vi "Keithley2100.ProcCases.vi"(0 "i ref in":refnum<vi>, 1 "selector":string, 2 "Data":T1, 3 "call cluster":T2={"Object"="", "Selector"="", "CallType"=enum."synchronous", "Async Object"="", "Async Selector"="", "Data Descriptor"="", "Data"=[], "Error #"=0, "Expire"=0}, 5 "error in (no error)":errorcluster) -> (14 "i ref out":refnum<vi>, 17 "answer cluster":T2={"Object"="", "Selector"="", "CallType"=enum."synchronous", "Async Object"="", "Async Selector"="", "Data Descriptor"="", "Data"=[], "Error #"=0, "Expire"=0}, 19 "error out":errorcluster)   [LabVIEW 2014, in "Keithley2100.lvlib"]
doc: "This method is called by a process from within the default case in the event loop. The methods of a class that are linked to events will be called from THIS method. Add your code here."
uses:
  Keithley2100.lvlib
  CS_Core/CSSystem/CoreDefs/CoreDefs.call_type.ctl
  CS_Core/BaseProcess/BaseProcess.descriptor string definition.ctl
  CS_Core/CSSystem/CoreDefs/CoreDefs.rawDataType.ctl
  CS_Core/CSSystem/CoreLib/CoreLib.string 2 byte array.vi
  CS_Core/CSSystem/CoreLib/CoreLib.double 2 byte array.vi
  CS_Core/CSSystem/CoreLib/CoreLib.byte array 2 int.vi
  CS_Core/CSSystem/CoreLib/CoreLib.byte array 2 double.vi
  CS_Core/CSSystem/CoreLib/CoreLib.lvlib
  CS_Core/BaseProcess/BaseProcess.lvlib
  CS_Core/CSApplicationBaseClasses/DeviceBase/DeviceBase.lvlib
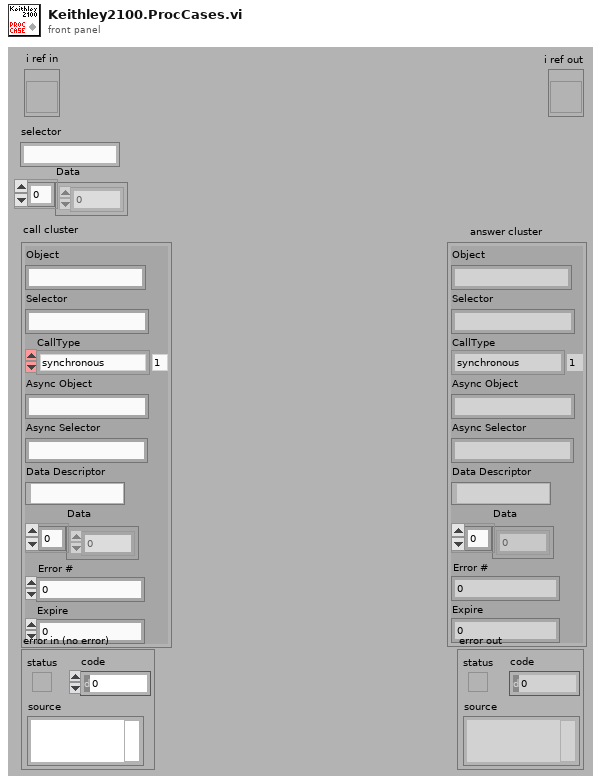
[diagram p1: front panel]
types:
  T1 = typedef "CoreDefs.rawDataType.ctl" = i8[]
  T2 = typedef "CoreDefs.call_type.ctl" = cluster{"Object":string, "Selector":string, "CallType":enum16{"simple", "synchronous", "asynchronous"}, "Async Object":string, "Async Selector":string, "Data Descriptor":T3, "Data":T1, "Error #":i32, "Expire":u32}
  T3 = typedef "BaseProcess.lvlib/BaseProcess.descriptor string definition.ctl" = string
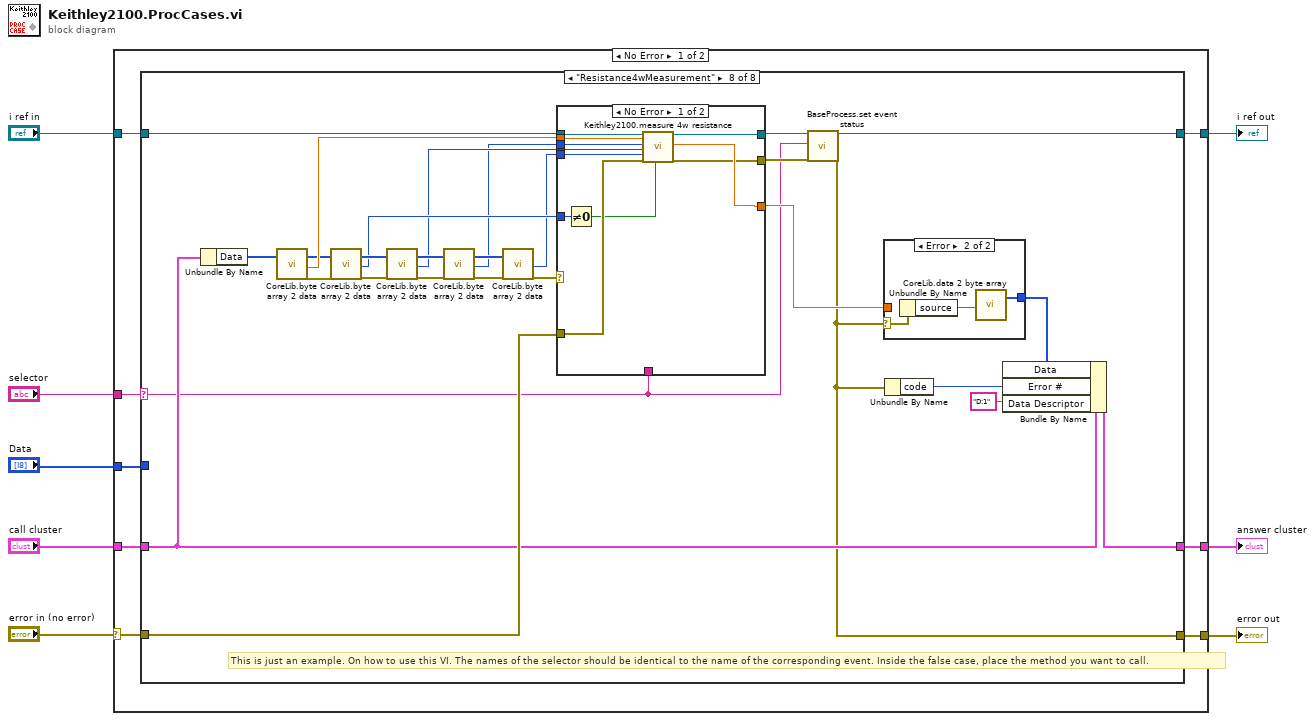
[diagram p0: block diagram]
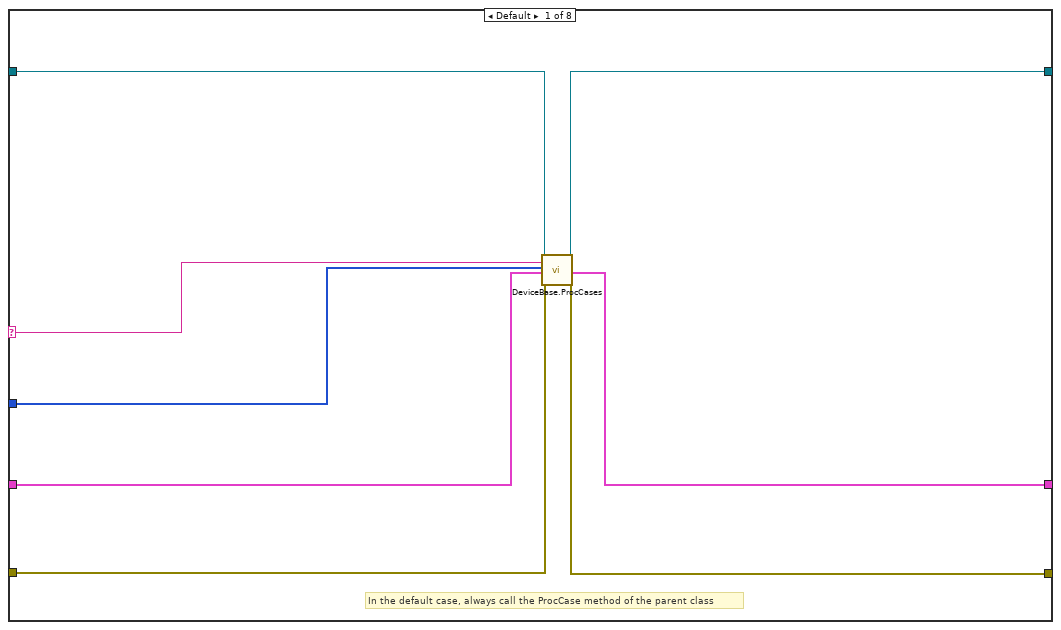
[diagram p2: hidden frame]
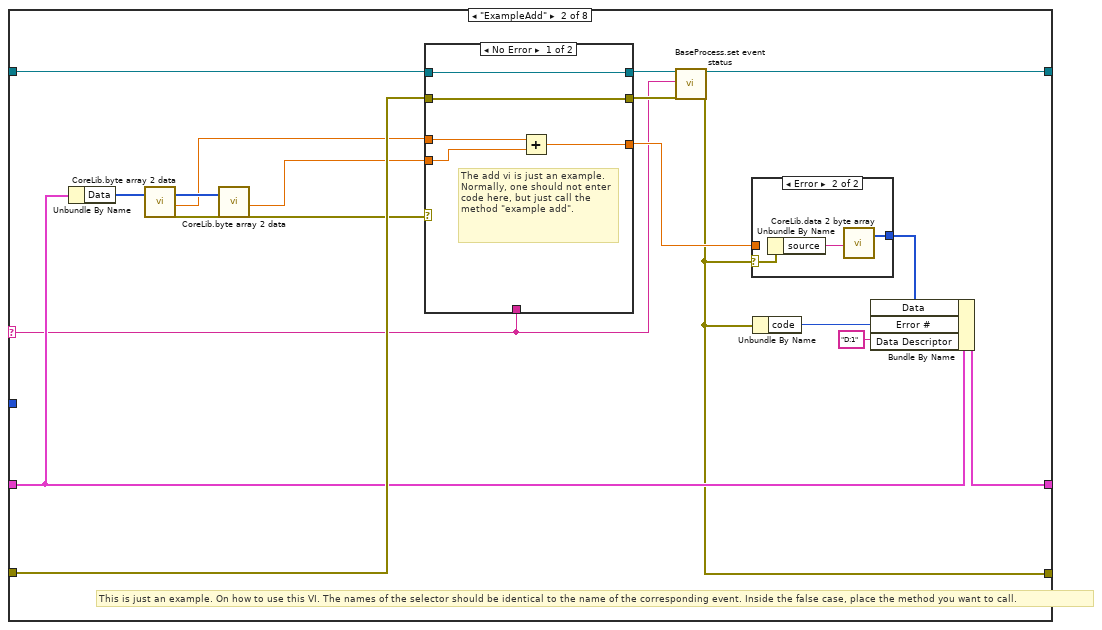
[diagram p3: hidden frame]
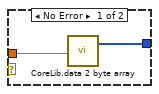
[diagram p4: hidden frame]
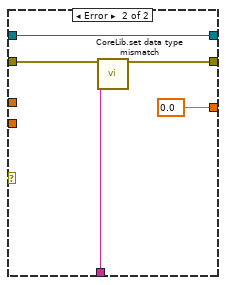
[diagram p5: hidden frame]
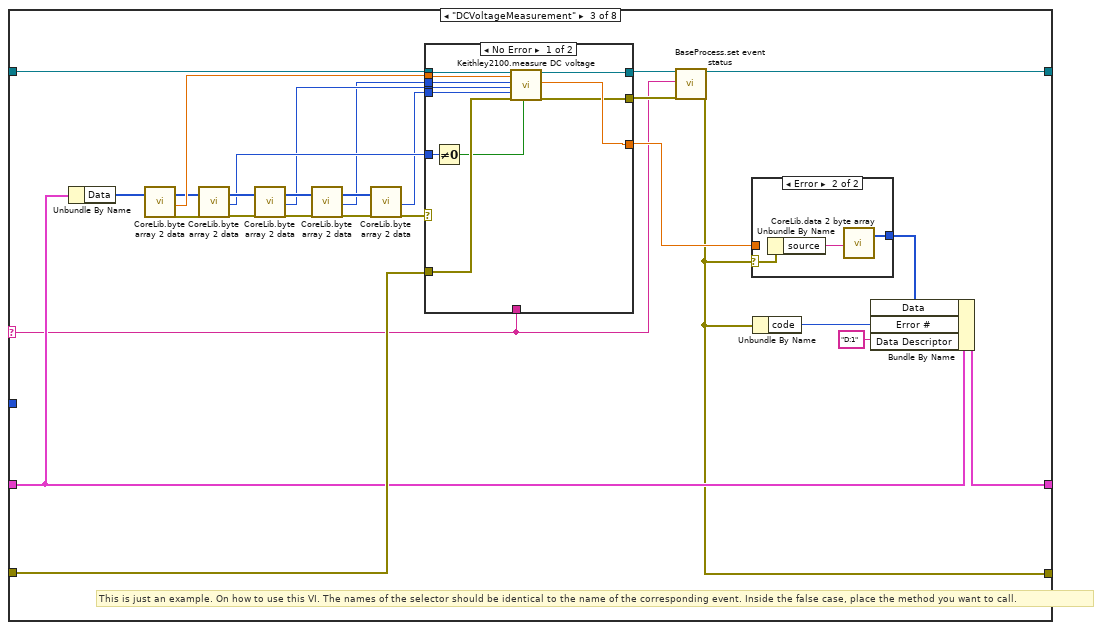
[diagram p6: hidden frame]
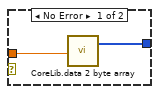
[diagram p7: hidden frame]
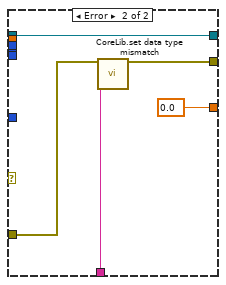
[diagram p8: hidden frame]
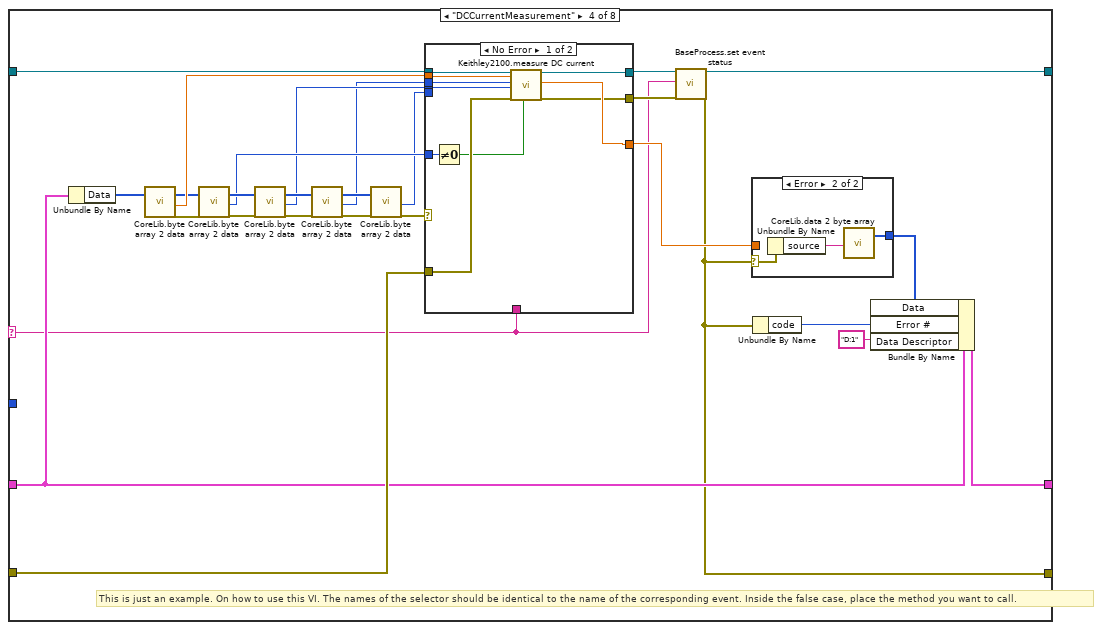
[diagram p9: hidden frame]
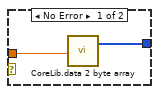
[diagram p10: hidden frame]
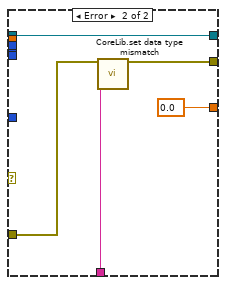
[diagram p11: hidden frame]
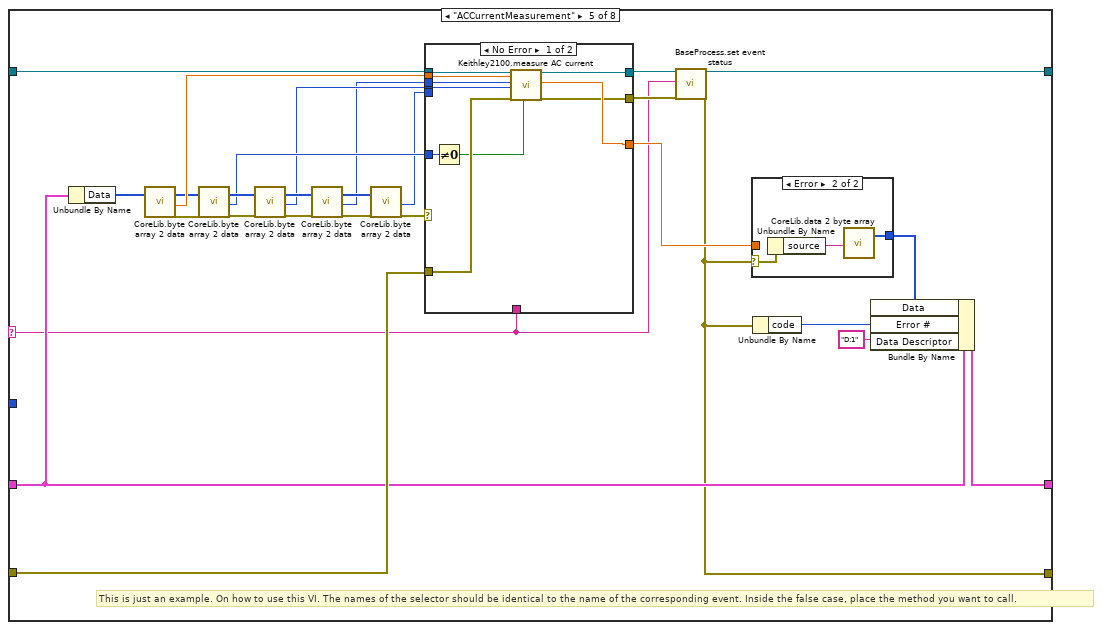
[diagram p12: hidden frame]
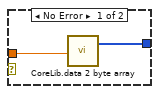
[diagram p13: hidden frame]
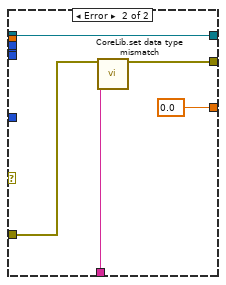
[diagram p14: hidden frame]
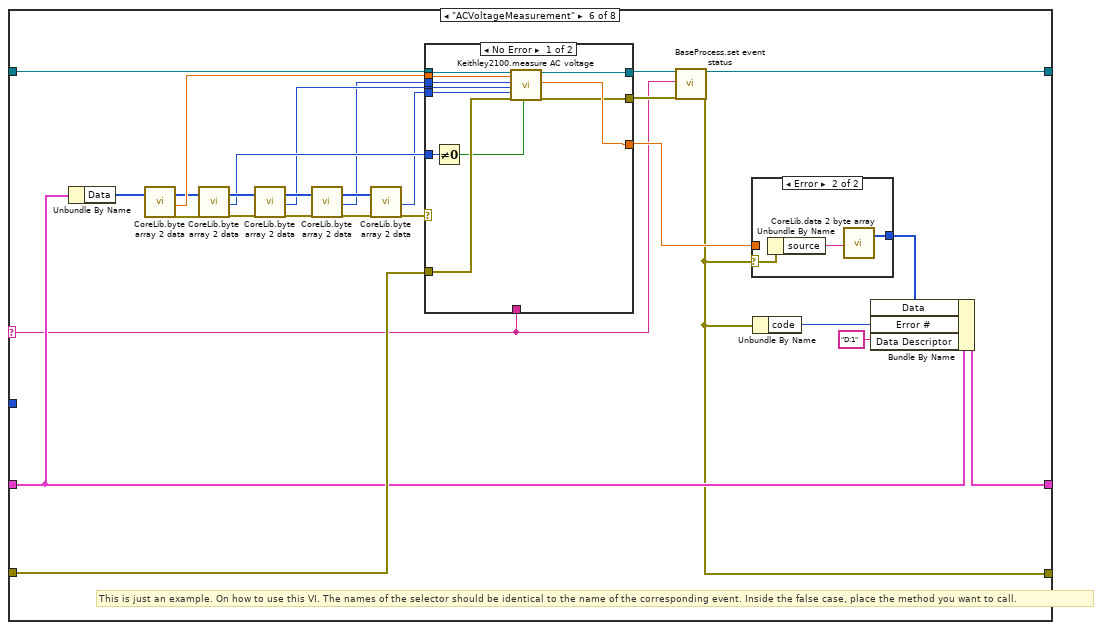
[diagram p15: hidden frame]
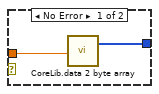
[diagram p16: hidden frame]
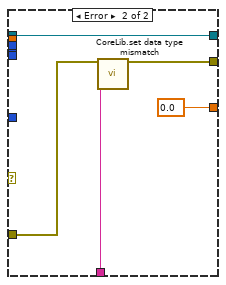
[diagram p17: hidden frame]
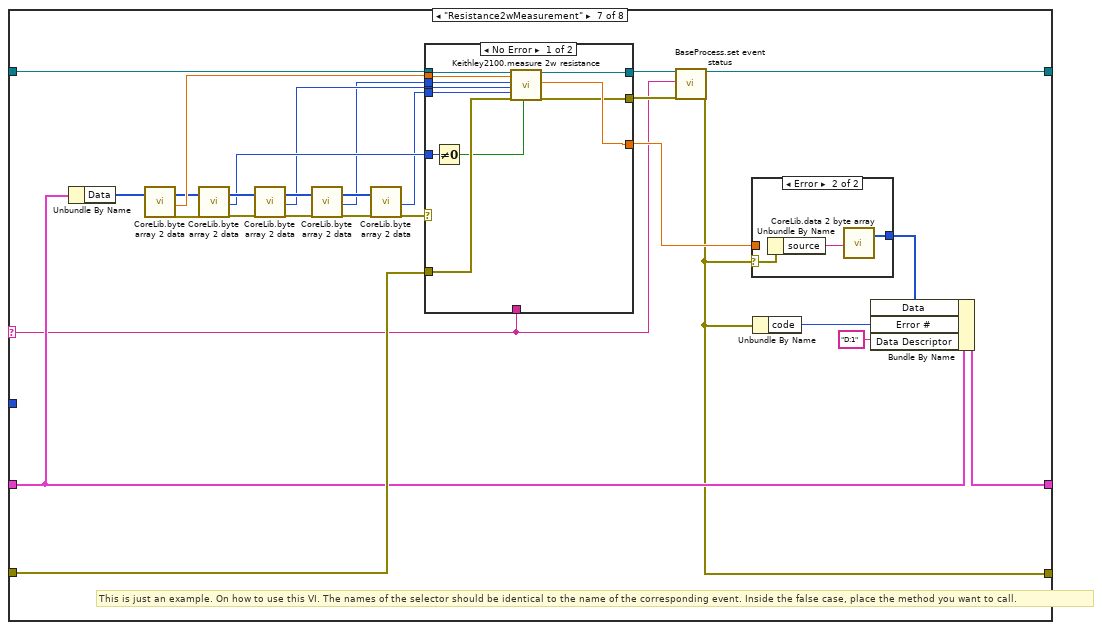
[diagram p18: hidden frame]
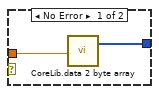
[diagram p19: hidden frame]
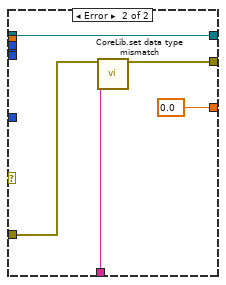
[diagram p20: hidden frame]
diagram:
  n1 = case shown="No Error" "error in (no error)" {
    selector: "error in (no error)" -> [w9 w351]
    tunnel: "selector" -> [w16 _]
    tunnel: [w15 w352] -> w7
    tunnel: "Data" -> [w14 _]
    tunnel: "call cluster" -> [w13 w352]
    tunnel: "i ref in" -> [w12 w353]
    tunnel: [w11 w353] -> w3
    tunnel: [w10 w351] -> w2
    frame No Error {
      n2 = case shown="\"Resistance4wMeasurement\"" w16 {
        selector: w16 -> [w19 w33 w76 w125 w173 w221 w270 w319]
        tunnel: w14 -> [w17 _ _ _ _ _ _ _]
        tunnel: w12 -> [w18 w43 w86 w135 w183 w231 w280 w329]
        tunnel: [w24 w32 w75 w124 w172 w220 w269 w318] -> w11
        tunnel: w13 -> [w20 w39 w82 w131 w179 w227 w276 w325]
        tunnel: [w21 w38 w81 w130 w178 w226 w275 w324] -> w15
        tunnel: w9 -> [w23 w42 w85 w134 w182 w230 w279 w328]
        tunnel: [w22 w34 w77 w126 w174 w222 w271 w320] -> w10
        frame Default {
          # "In the default case, always call the ProcCase method of the parent class"
          n3 = call "DeviceBase.ProcCases.vi"("i ref in"=w18, "selector"=w19, "Data"=w17, "call cluster"=w20, "error in (no error)"=w23) -> ("i ref out"=w24:refnum<vi>, "answer cluster"=w21:T2, "error out"=w22:errorcluster)  [unwired: 12 in]
        }
        frame "ExampleAdd" {
          # "This is just an example. On how to use this VI. The names of the selector should be identical to the name of the corresponding event. Inside the false case, place the method you want to call."
          n4 = Unbundle By Name(w39) -> ("Data"=w30:T1)
          n5 = call-poly "CoreLib.byte array 2 data.vi"("byteArray"=w30) -> ("byteArray out"=w28:T1, "d64"=w26:dbl, "error out"=w29:errorcluster)  [unwired: 16 in]
          n6 = call-poly "CoreLib.byte array 2 data.vi"("byteArray"=w28, "error in (no error)"=w29) -> ("d64"=w25:dbl, "error out"=w27:errorcluster)  [unwired: 15 in, 1 out]
          n7 = case shown="No Error" w27 {
            tunnel: [w50 w58] -> w36
            tunnel: w43 -> [w50 w58]
            tunnel: w42 -> [w51 w57]
            tunnel: [w51 w56] -> w35
            tunnel: w25 -> [w53 _]
            tunnel: [w52 0.0] -> w41
            tunnel: w33 -> [_ w54]
            tunnel: w26 -> [w49 _]
            frame No Error {
              # "The add vi is just an example. Normally, one should not enter code here, but just call the method \"example add\"."
              n8 = Add(x=w49, y=w53) -> (x+y=w52:dbl)
            }
            frame Error {
              n9 = call "CoreLib.set data type mismatch.vi"("error in (no error)"=w57, "error source"=w54) -> ("error out"=w56:errorcluster)  [unwired: 17 in]
            }
          }
          n10 = call "BaseProcess.set event status.vi"("i ref in"=w36, "EventStatus"=w33, "error in (no error)"=w35) -> ("i ref out"=w32:refnum<vi>, "error out"=w34:errorcluster)  [unwired: 14 in, 1 out]
          n11 = case shown="Error" w34 {
            selector: w34 -> [_ w48]
            tunnel: [w44 w47] -> w37
            tunnel: w41 -> [w45 _]
            frame No Error {
              n12 = call-poly "CoreLib.data 2 byte array.vi"("f64"=w45) -> ("byteArray out"=w44:T1)  [unwired: 18 in]
            }
            frame Error {
              n13 = Unbundle By Name(w48) -> ("source"=w46:string)
              n14 = call-poly "CoreLib.data 2 byte array.vi"("string"=w46) -> ("byteArray out"=w47:T1)  [unwired: 18 in]
            }
          }
          n15 = Unbundle By Name(w34) -> ("code"=w40:i32)
          n16 = Bundle By Name(cluster=w39, "Data"=w37, "Error #"=w40, "Data Descriptor"="D:1") -> (w38:T2)
        }
        frame "DCVoltageMeasurement" {
          # "This is just an example. On how to use this VI. The names of the selector should be identical to the name of the corresponding event. Inside the false case, place the method you want to call."
          n17 = Unbundle By Name(w82) -> ("Data"=w73:T1)
          n18 = call-poly "CoreLib.byte array 2 data.vi"("byteArray"=w73) -> ("byteArray out"=w71:T1, "d64"=w72:dbl, "error out"=w70:errorcluster)  [unwired: 16 in]
          n19 = call-poly "CoreLib.byte array 2 data.vi"("byteArray"=w71, "error in (no error)"=w70) -> ("byteArray out"=w69:T1, "i32"=w62:i32, "error out"=w66:errorcluster)  [unwired: 15 in]
          n20 = call-poly "CoreLib.byte array 2 data.vi"("byteArray"=w69, "error in (no error)"=w66) -> ("byteArray out"=w68:T1, "i32"=w61:i32, "error out"=w65:errorcluster)  [unwired: 15 in]
          n21 = call-poly "CoreLib.byte array 2 data.vi"("byteArray"=w68, "error in (no error)"=w65) -> ("byteArray out"=w67:T1, "i32"=w60:i32, "error out"=w64:errorcluster)  [unwired: 15 in]
          n22 = call-poly "CoreLib.byte array 2 data.vi"("byteArray"=w67, "error in (no error)"=w64) -> ("i32"=w59:i32, "error out"=w63:errorcluster)  [unwired: 15 in, 1 out]
          n23 = case shown="No Error" w63 {
            tunnel: [w101 w107] -> w79
            tunnel: w86 -> [w102 w107]
            tunnel: w85 -> [w98 w106]
            tunnel: [w99 w105] -> w78
            tunnel: [w100 0.0] -> w84
            tunnel: w76 -> [_ w103]
            tunnel: w72 -> [w97 _]
            tunnel: w62 -> [w96 _]
            tunnel: w61 -> [w94 _]
            tunnel: w60 -> [w93 _]
            tunnel: w59 -> [w92 _]
            frame No Error {
              n24 = Not Equal To 0?(x=w96) -> (x != 0?=w95:bool)
              n25 = call "Keithley2100.measure DC voltage.vi"("i ref in"=w102, "Custom Range (100mV)"=w97, "Digital Filter (0: Off)"=w93, "Digital Filter Readings (10)"=w94, "NPLC"=w92, "error in (no error)"=w98, "Auto Range"=w95) -> ("i refout"=w101:refnum<vi>, "Measurement"=w100:dbl, "error out"=w99:errorcluster)  [unwired: 10 in]
            }
            frame Error {
              n26 = call "CoreLib.set data type mismatch.vi"("error in (no error)"=w106, "error source"=w103) -> ("error out"=w105:errorcluster)  [unwired: 17 in]
            }
          }
          n27 = call "BaseProcess.set event status.vi"("i ref in"=w79, "EventStatus"=w76, "error in (no error)"=w78) -> ("i ref out"=w75:refnum<vi>, "error out"=w77:errorcluster)  [unwired: 14 in, 1 out]
          n28 = case shown="Error" w77 {
            selector: w77 -> [_ w91]
            tunnel: [w87 w90] -> w80
            tunnel: w84 -> [w88 _]
            frame No Error {
              n29 = call-poly "CoreLib.data 2 byte array.vi"("f64"=w88) -> ("byteArray out"=w87:T1)  [unwired: 18 in]
            }
            frame Error {
              n30 = Unbundle By Name(w91) -> ("source"=w89:string)
              n31 = call-poly "CoreLib.data 2 byte array.vi"("string"=w89) -> ("byteArray out"=w90:T1)  [unwired: 18 in]
            }
          }
          n32 = Unbundle By Name(w77) -> ("code"=w83:i32)
          n33 = Bundle By Name(cluster=w82, "Data"=w80, "Error #"=w83, "Data Descriptor"="D:1") -> (w81:T2)
        }
        frame "DCCurrentMeasurement" {
          # "This is just an example. On how to use this VI. The names of the selector should be identical to the name of the corresponding event. Inside the false case, place the method you want to call."
          n34 = Unbundle By Name(w131) -> ("Data"=w122:T1)
          n35 = call-poly "CoreLib.byte array 2 data.vi"("byteArray"=w122) -> ("byteArray out"=w120:T1, "d64"=w121:dbl, "error out"=w119:errorcluster)  [unwired: 16 in]
          n36 = call-poly "CoreLib.byte array 2 data.vi"("byteArray"=w120, "error in (no error)"=w119) -> ("byteArray out"=w118:T1, "i32"=w111:i32, "error out"=w115:errorcluster)  [unwired: 15 in]
          n37 = call-poly "CoreLib.byte array 2 data.vi"("byteArray"=w118, "error in (no error)"=w115) -> ("byteArray out"=w117:T1, "i32"=w110:i32, "error out"=w114:errorcluster)  [unwired: 15 in]
          n38 = call-poly "CoreLib.byte array 2 data.vi"("byteArray"=w117, "error in (no error)"=w114) -> ("byteArray out"=w116:T1, "i32"=w109:i32, "error out"=w113:errorcluster)  [unwired: 15 in]
          n39 = call-poly "CoreLib.byte array 2 data.vi"("byteArray"=w116, "error in (no error)"=w113) -> ("i32"=w108:i32, "error out"=w112:errorcluster)  [unwired: 15 in, 1 out]
          n40 = case shown="No Error" w112 {
            tunnel: [w149 w155] -> w128
            tunnel: w135 -> [w150 w155]
            tunnel: w134 -> [w146 w154]
            tunnel: [w147 w153] -> w127
            tunnel: [w148 0.0] -> w133
            tunnel: w125 -> [_ w151]
            tunnel: w121 -> [w145 _]
            tunnel: w111 -> [w144 _]
            tunnel: w110 -> [w142 _]
            tunnel: w109 -> [w141 _]
            tunnel: w108 -> [_ _]
            frame No Error {
              n41 = Not Equal To 0?(x=w144) -> (x != 0?=w143:bool)
              n42 = call "Keithley2100.measure DC current.vi"("i ref in"=w150, "Custom Range (0 A)"=w145, "Digital Filter (0: Off)"=w141, "Digital Filter Readings (10)"=w142, "error in (no error)"=w146, "Auto Range"=w143) -> ("i refout"=w149:refnum<vi>, "Measurement"=w148:dbl, "error out"=w147:errorcluster)  [unwired: 11 in]
            }
            frame Error {
              n43 = call "CoreLib.set data type mismatch.vi"("error in (no error)"=w154, "error source"=w151) -> ("error out"=w153:errorcluster)  [unwired: 17 in]
            }
          }
          n44 = call "BaseProcess.set event status.vi"("i ref in"=w128, "EventStatus"=w125, "error in (no error)"=w127) -> ("i ref out"=w124:refnum<vi>, "error out"=w126:errorcluster)  [unwired: 14 in, 1 out]
          n45 = case shown="Error" w126 {
            selector: w126 -> [_ w140]
            tunnel: [w136 w139] -> w129
            tunnel: w133 -> [w137 _]
            frame No Error {
              n46 = call-poly "CoreLib.data 2 byte array.vi"("f64"=w137) -> ("byteArray out"=w136:T1)  [unwired: 18 in]
            }
            frame Error {
              n47 = Unbundle By Name(w140) -> ("source"=w138:string)
              n48 = call-poly "CoreLib.data 2 byte array.vi"("string"=w138) -> ("byteArray out"=w139:T1)  [unwired: 18 in]
            }
          }
          n49 = Unbundle By Name(w126) -> ("code"=w132:i32)
          n50 = Bundle By Name(cluster=w131, "Data"=w129, "Error #"=w132, "Data Descriptor"="D:1") -> (w130:T2)
        }
        frame "ACCurrentMeasurement" {
          # "This is just an example. On how to use this VI. The names of the selector should be identical to the name of the corresponding event. Inside the false case, place the method you want to call."
          n51 = Unbundle By Name(w179) -> ("Data"=w170:T1)
          n52 = call-poly "CoreLib.byte array 2 data.vi"("byteArray"=w170) -> ("byteArray out"=w168:T1, "d64"=w169:dbl, "error out"=w167:errorcluster)  [unwired: 16 in]
          n53 = call-poly "CoreLib.byte array 2 data.vi"("byteArray"=w168, "error in (no error)"=w167) -> ("byteArray out"=w166:T1, "i32"=w159:i32, "error out"=w163:errorcluster)  [unwired: 15 in]
          n54 = call-poly "CoreLib.byte array 2 data.vi"("byteArray"=w166, "error in (no error)"=w163) -> ("byteArray out"=w165:T1, "i32"=w158:i32, "error out"=w162:errorcluster)  [unwired: 15 in]
          n55 = call-poly "CoreLib.byte array 2 data.vi"("byteArray"=w165, "error in (no error)"=w162) -> ("byteArray out"=w164:T1, "i32"=w157:i32, "error out"=w161:errorcluster)  [unwired: 15 in]
          n56 = call-poly "CoreLib.byte array 2 data.vi"("byteArray"=w164, "error in (no error)"=w161) -> ("i32"=w156:i32, "error out"=w160:errorcluster)  [unwired: 15 in, 1 out]
          n57 = case shown="No Error" w160 {
            tunnel: [w197 w203] -> w176
            tunnel: w183 -> [w198 w203]
            tunnel: w182 -> [w194 w202]
            tunnel: [w195 w201] -> w175
            tunnel: [w196 0.0] -> w181
            tunnel: w173 -> [_ w199]
            tunnel: w169 -> [w193 _]
            tunnel: w159 -> [w192 _]
            tunnel: w158 -> [w190 _]
            tunnel: w157 -> [w189 _]
            tunnel: w156 -> [_ _]
            frame No Error {
              n58 = Not Equal To 0?(x=w192) -> (x != 0?=w191:bool)
              n59 = call "Keithley2100.measure AC current.vi"("i ref in"=w198, "Custom Range (100mV)"=w193, "Digital Filter (0: Off)"=w189, "Digital Filter Readings (10)"=w190, "error in (no error)"=w194, "Auto Range"=w191) -> ("i refout"=w197:refnum<vi>, "Measurement"=w196:dbl, "error out"=w195:errorcluster)  [unwired: 11 in]
            }
            frame Error {
              n60 = call "CoreLib.set data type mismatch.vi"("error in (no error)"=w202, "error source"=w199) -> ("error out"=w201:errorcluster)  [unwired: 17 in]
            }
          }
          n61 = call "BaseProcess.set event status.vi"("i ref in"=w176, "EventStatus"=w173, "error in (no error)"=w175) -> ("i ref out"=w172:refnum<vi>, "error out"=w174:errorcluster)  [unwired: 14 in, 1 out]
          n62 = case shown="Error" w174 {
            selector: w174 -> [_ w188]
            tunnel: [w184 w187] -> w177
            tunnel: w181 -> [w185 _]
            frame No Error {
              n63 = call-poly "CoreLib.data 2 byte array.vi"("f64"=w185) -> ("byteArray out"=w184:T1)  [unwired: 18 in]
            }
            frame Error {
              n64 = Unbundle By Name(w188) -> ("source"=w186:string)
              n65 = call-poly "CoreLib.data 2 byte array.vi"("string"=w186) -> ("byteArray out"=w187:T1)  [unwired: 18 in]
            }
          }
          n66 = Unbundle By Name(w174) -> ("code"=w180:i32)
          n67 = Bundle By Name(cluster=w179, "Data"=w177, "Error #"=w180, "Data Descriptor"="D:1") -> (w178:T2)
        }
        frame "ACVoltageMeasurement" {
          # "This is just an example. On how to use this VI. The names of the selector should be identical to the name of the corresponding event. Inside the false case, place the method you want to call."
          n68 = Unbundle By Name(w227) -> ("Data"=w218:T1)
          n69 = call-poly "CoreLib.byte array 2 data.vi"("byteArray"=w218) -> ("byteArray out"=w216:T1, "d64"=w217:dbl, "error out"=w215:errorcluster)  [unwired: 16 in]
          n70 = call-poly "CoreLib.byte array 2 data.vi"("byteArray"=w216, "error in (no error)"=w215) -> ("byteArray out"=w214:T1, "i32"=w207:i32, "error out"=w211:errorcluster)  [unwired: 15 in]
          n71 = call-poly "CoreLib.byte array 2 data.vi"("byteArray"=w214, "error in (no error)"=w211) -> ("byteArray out"=w213:T1, "i32"=w206:i32, "error out"=w210:errorcluster)  [unwired: 15 in]
          n72 = call-poly "CoreLib.byte array 2 data.vi"("byteArray"=w213, "error in (no error)"=w210) -> ("byteArray out"=w212:T1, "i32"=w205:i32, "error out"=w209:errorcluster)  [unwired: 15 in]
          n73 = call-poly "CoreLib.byte array 2 data.vi"("byteArray"=w212, "error in (no error)"=w209) -> ("i32"=w204:i32, "error out"=w208:errorcluster)  [unwired: 15 in, 1 out]
          n74 = case shown="No Error" w208 {
            tunnel: [w246 w252] -> w224
            tunnel: w231 -> [w247 w252]
            tunnel: w230 -> [w243 w251]
            tunnel: [w244 w250] -> w223
            tunnel: [w245 0.0] -> w229
            tunnel: w221 -> [_ w248]
            tunnel: w217 -> [w242 _]
            tunnel: w207 -> [w241 _]
            tunnel: w206 -> [w239 _]
            tunnel: w205 -> [w238 _]
            tunnel: w204 -> [w237 _]
            frame No Error {
              n75 = Not Equal To 0?(x=w241) -> (x != 0?=w240:bool)
              n76 = call "Keithley2100.measure AC voltage.vi"("i ref in"=w247, "Custom Range (100mV)"=w242, "Digital Filter (0: Off)"=w238, "Digital Filter Readings (10)"=w239, "NPLC"=w237, "error in (no error)"=w243, "Auto Range"=w240) -> ("i refout"=w246:refnum<vi>, "Measurement"=w245:dbl, "error out"=w244:errorcluster)  [unwired: 10 in]
            }
            frame Error {
              n77 = call "CoreLib.set data type mismatch.vi"("error in (no error)"=w251, "error source"=w248) -> ("error out"=w250:errorcluster)  [unwired: 17 in]
            }
          }
          n78 = call "BaseProcess.set event status.vi"("i ref in"=w224, "EventStatus"=w221, "error in (no error)"=w223) -> ("i ref out"=w220:refnum<vi>, "error out"=w222:errorcluster)  [unwired: 14 in, 1 out]
          n79 = case shown="Error" w222 {
            selector: w222 -> [_ w236]
            tunnel: [w232 w235] -> w225
            tunnel: w229 -> [w233 _]
            frame No Error {
              n80 = call-poly "CoreLib.data 2 byte array.vi"("f64"=w233) -> ("byteArray out"=w232:T1)  [unwired: 18 in]
            }
            frame Error {
              n81 = Unbundle By Name(w236) -> ("source"=w234:string)
              n82 = call-poly "CoreLib.data 2 byte array.vi"("string"=w234) -> ("byteArray out"=w235:T1)  [unwired: 18 in]
            }
          }
          n83 = Unbundle By Name(w222) -> ("code"=w228:i32)
          n84 = Bundle By Name(cluster=w227, "Data"=w225, "Error #"=w228, "Data Descriptor"="D:1") -> (w226:T2)
        }
        frame "Resistance2wMeasurement" {
          # "This is just an example. On how to use this VI. The names of the selector should be identical to the name of the corresponding event. Inside the false case, place the method you want to call."
          n85 = Unbundle By Name(w276) -> ("Data"=w267:T1)
          n86 = call-poly "CoreLib.byte array 2 data.vi"("byteArray"=w267) -> ("byteArray out"=w265:T1, "d64"=w266:dbl, "error out"=w264:errorcluster)  [unwired: 16 in]
          n87 = call-poly "CoreLib.byte array 2 data.vi"("byteArray"=w265, "error in (no error)"=w264) -> ("byteArray out"=w263:T1, "i32"=w256:i32, "error out"=w260:errorcluster)  [unwired: 15 in]
          n88 = call-poly "CoreLib.byte array 2 data.vi"("byteArray"=w263, "error in (no error)"=w260) -> ("byteArray out"=w262:T1, "i32"=w255:i32, "error out"=w259:errorcluster)  [unwired: 15 in]
          n89 = call-poly "CoreLib.byte array 2 data.vi"("byteArray"=w262, "error in (no error)"=w259) -> ("byteArray out"=w261:T1, "i32"=w254:i32, "error out"=w258:errorcluster)  [unwired: 15 in]
          n90 = call-poly "CoreLib.byte array 2 data.vi"("byteArray"=w261, "error in (no error)"=w258) -> ("i32"=w253:i32, "error out"=w257:errorcluster)  [unwired: 15 in, 1 out]
          n91 = case shown="No Error" w257 {
            tunnel: [w295 w301] -> w273
            tunnel: w280 -> [w296 w301]
            tunnel: w279 -> [w292 w300]
            tunnel: [w293 w299] -> w272
            tunnel: [w294 0.0] -> w278
            tunnel: w270 -> [_ w297]
            tunnel: w266 -> [w291 _]
            tunnel: w256 -> [w290 _]
            tunnel: w255 -> [w288 _]
            tunnel: w254 -> [w287 _]
            tunnel: w253 -> [w286 _]
            frame No Error {
              n92 = Not Equal To 0?(x=w290) -> (x != 0?=w289:bool)
              n93 = call "Keithley2100.measure 2w resistance.vi"("i ref in"=w296, "Custom Range (100mV)"=w291, "Digital Filter (0: Off)"=w287, "Digital Filter Readings (10)"=w288, "NPLC"=w286, "error in (no error)"=w292, "Auto Range"=w289) -> ("i refout"=w295:refnum<vi>, "Measurement"=w294:dbl, "error out"=w293:errorcluster)  [unwired: 10 in]
            }
            frame Error {
              n94 = call "CoreLib.set data type mismatch.vi"("error in (no error)"=w300, "error source"=w297) -> ("error out"=w299:errorcluster)  [unwired: 17 in]
            }
          }
          n95 = call "BaseProcess.set event status.vi"("i ref in"=w273, "EventStatus"=w270, "error in (no error)"=w272) -> ("i ref out"=w269:refnum<vi>, "error out"=w271:errorcluster)  [unwired: 14 in, 1 out]
          n96 = case shown="Error" w271 {
            selector: w271 -> [_ w285]
            tunnel: [w281 w284] -> w274
            tunnel: w278 -> [w282 _]
            frame No Error {
              n97 = call-poly "CoreLib.data 2 byte array.vi"("f64"=w282) -> ("byteArray out"=w281:T1)  [unwired: 18 in]
            }
            frame Error {
              n98 = Unbundle By Name(w285) -> ("source"=w283:string)
              n99 = call-poly "CoreLib.data 2 byte array.vi"("string"=w283) -> ("byteArray out"=w284:T1)  [unwired: 18 in]
            }
          }
          n100 = Unbundle By Name(w271) -> ("code"=w277:i32)
          n101 = Bundle By Name(cluster=w276, "Data"=w274, "Error #"=w277, "Data Descriptor"="D:1") -> (w275:T2)
        }
        frame "Resistance4wMeasurement" {
          # "This is just an example. On how to use this VI. The names of the selector should be identical to the name of the corresponding event. Inside the false case, place the method you want to call."
          n102 = Unbundle By Name(w325) -> ("Data"=w316:T1)
          n103 = call-poly "CoreLib.byte array 2 data.vi"("byteArray"=w316) -> ("byteArray out"=w314:T1, "d64"=w315:dbl, "error out"=w313:errorcluster)  [unwired: 16 in]
          n104 = call-poly "CoreLib.byte array 2 data.vi"("byteArray"=w314, "error in (no error)"=w313) -> ("byteArray out"=w312:T1, "i32"=w305:i32, "error out"=w309:errorcluster)  [unwired: 15 in]
          n105 = call-poly "CoreLib.byte array 2 data.vi"("byteArray"=w312, "error in (no error)"=w309) -> ("byteArray out"=w311:T1, "i32"=w304:i32, "error out"=w308:errorcluster)  [unwired: 15 in]
          n106 = call-poly "CoreLib.byte array 2 data.vi"("byteArray"=w311, "error in (no error)"=w308) -> ("byteArray out"=w310:T1, "i32"=w303:i32, "error out"=w307:errorcluster)  [unwired: 15 in]
          n107 = call-poly "CoreLib.byte array 2 data.vi"("byteArray"=w310, "error in (no error)"=w307) -> ("i32"=w302:i32, "error out"=w306:errorcluster)  [unwired: 15 in, 1 out]
          n108 = case shown="No Error" w306 {
            tunnel: [w344 w350] -> w322
            tunnel: w329 -> [w345 w350]
            tunnel: w328 -> [w341 w349]
            tunnel: [w342 w348] -> w321
            tunnel: [w343 0.0] -> w327
            tunnel: w319 -> [_ w346]
            tunnel: w315 -> [w340 _]
            tunnel: w305 -> [w339 _]
            tunnel: w304 -> [w337 _]
            tunnel: w303 -> [w336 _]
            tunnel: w302 -> [w335 _]
            frame No Error {
              n109 = Not Equal To 0?(x=w339) -> (x != 0?=w338:bool)
              n110 = call "Keithley2100.measure 4w resistance.vi"("i ref in"=w345, "Custom Range (100mV)"=w340, "Digital Filter (0: Off)"=w336, "Digital Filter Readings (10)"=w337, "NPLC"=w335, "error in (no error)"=w341, "Auto Range"=w338) -> ("i refout"=w344:refnum<vi>, "Measurement"=w343:dbl, "error out"=w342:errorcluster)  [unwired: 10 in]
            }
            frame Error {
              n111 = call "CoreLib.set data type mismatch.vi"("error in (no error)"=w349, "error source"=w346) -> ("error out"=w348:errorcluster)  [unwired: 17 in]
            }
          }
          n112 = call "BaseProcess.set event status.vi"("i ref in"=w322, "EventStatus"=w319, "error in (no error)"=w321) -> ("i ref out"=w318:refnum<vi>, "error out"=w320:errorcluster)  [unwired: 14 in, 1 out]
          n113 = case shown="Error" w320 {
            selector: w320 -> [_ w334]
            tunnel: [w330 w333] -> w323
            tunnel: w327 -> [w331 _]
            frame No Error {
              n114 = call-poly "CoreLib.data 2 byte array.vi"("f64"=w331) -> ("byteArray out"=w330:T1)  [unwired: 18 in]
            }
            frame Error {
              n115 = Unbundle By Name(w334) -> ("source"=w332:string)
              n116 = call-poly "CoreLib.data 2 byte array.vi"("string"=w332) -> ("byteArray out"=w333:T1)  [unwired: 18 in]
            }
          }
          n117 = Unbundle By Name(w320) -> ("code"=w326:i32)
          n118 = Bundle By Name(cluster=w325, "Data"=w323, "Error #"=w326, "Data Descriptor"="D:1") -> (w324:T2)
        }
      }
    }
    frame Error {
    }
  }
  "answer cluster" <- w7
  "i ref out" <- w3
  "error out" <- w2
